vi "Stop API.vi"(8 "Error In":errorcluster) -> (0 "Error Out":errorcluster)   [LabVIEW 2017, in "Scope.lvlib"]
uses:
  Scope.lvlib
  Controls/Command Data [cluster].ctl
  Controls/Commands [enum].ctl
  Events/Events.lvlib
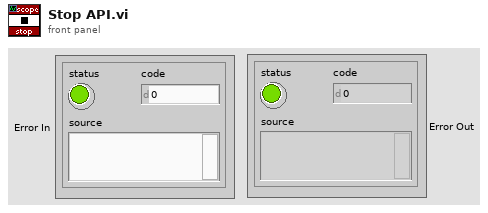
[diagram p1: front panel]
types:
  T1 = typedef "Scope.lvlib/Command Data [cluster].ctl" = cluster{"Command":T2, "Data":variant}
  T2 = typedef "Scope.lvlib/Commands [enum].ctl" = enum16{"Calculate parameters", "Start", "Stop", "Send data", "Start acquisition", "Get test data", "Accumulate test data", "Average test data", "Add background voltage", "Scale TPC", "Average Pre Trigger Data", "Write to file"}
  T3 = typedef "Events.lvlib/Refs [cluster].ctl" = cluster{"Exit":refnum<user-event>, "Controller":refnum<user-event>, "System Error":refnum<user-event>, "UI":refnum<user-event>, "Example Module":refnum<user-event>, "Shutter":refnum<user-event>, "Monochromator":refnum<user-event>, "DAQ":refnum<user-event>, "Scope":refnum<user-event>, "Processing":refnum<user-event>, "File IO":refnum<user-event>, "Colour wheel":refnum<user-event>}
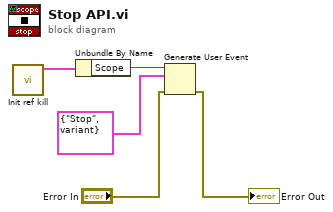
[diagram p0: block diagram]
diagram:
  n1 = call "Init ref kill.vi"() -> ("Messages"=w5:T3)  [unwired: 10 in, 1 out]
  n2 = Unbundle By Name(w5) -> ("Scope"=w4:refnum<user-event>)
  n3 = Generate User Event(user event=w4, event data cluster=T1 {"Command"=enum."Stop", "Data"=variant} ("event data"), error in="Error In") -> (error out=→"Error Out":errorcluster)  [unwired: 1 in, 1 out]
